vi "Execute.vi"(5 "user event in 2":refnum<user-event>, 7 "user event in":refnum<user-event>, 8 "Advanced Waveform In":refnum<class "Advanced Waveform.lvclass">, 9 "Set Frequency Message in":refnum<class "Set Frequency Message.lvclass">, 10 "Command Queue":refnum<queue>, 11 "error in (no error)":errorcluster) -> (0 "Advanced Waveform Out":refnum<class "Advanced Waveform.lvclass">, 1 "Set Frequency Message out":refnum<class "Set Frequency Message.lvclass">, 2 "Stop":bool, 3 "error out":errorcluster)   [LabVIEW 2011, in "Set Frequency Message.lvclass"]
uses:
  Set Frequency Message.lvclass
  Advanced Waveform Class/Advanced Waveform.lvclass
  Message.lvclass
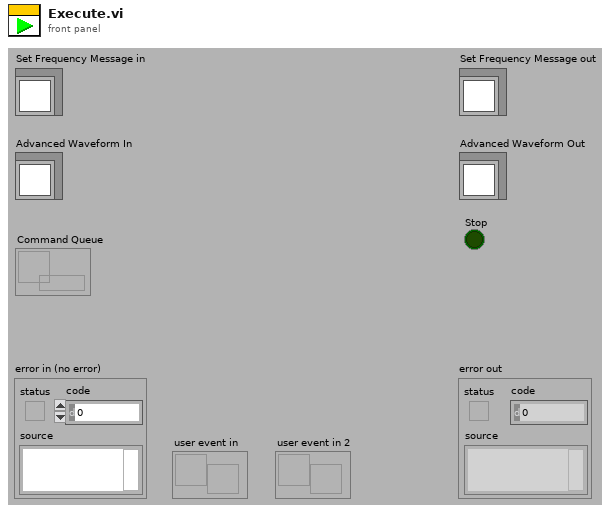
[diagram p1: front panel]
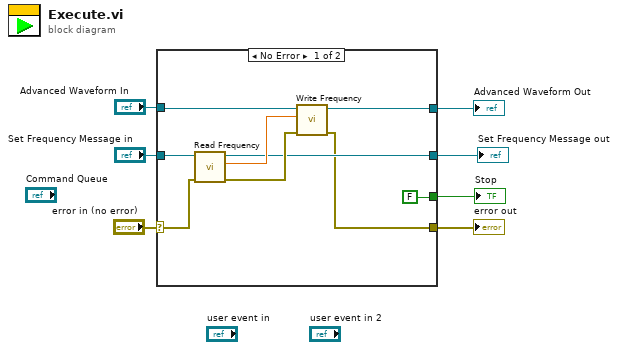
[diagram p0: block diagram]
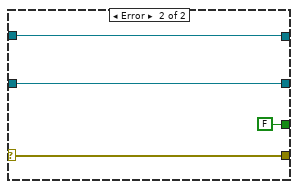
[diagram p2: hidden frame]
diagram:
  n1 = case shown="No Error" "error in (no error)" {
    selector: "error in (no error)" -> [w9 w17]
    tunnel: [w8 w17] -> w6
    tunnel: "Advanced Waveform In" -> [w15 w20]
    tunnel: "Set Frequency Message in" -> [w16 w19]
    tunnel: [w12 w19] -> w3
    tunnel: [w11 w20] -> w2
    tunnel: [FALSE FALSE] -> w1
    frame No Error {
      n2 = call-dynamic "Read Frequency.vi"("error in (no error)"=w9, "Set Frequency Message in"=w16) -> ("error out"=w13:errorcluster, "Frequency"=w14:dbl, "Set Frequency Message out"=w12:refnum<class "Set Frequency Message.lvclass">)  [unwired: 7 in]
      n3 = call-dynamic "Write Frequency.vi"("error in (no error)"=w13, "Frequency"=w14, "Waveform in"=w15) -> ("error out"=w8:errorcluster, "Waveform out"=w11:refnum<class "Advanced Waveform.lvclass">)  [unwired: 7 in]
    }
    frame Error {
    }
  }
  "error out" <- w6
  "Set Frequency Message out" <- w3
  "Stop" <- w1
  "Advanced Waveform Out" <- w2
